vi "Process Monitor.vi"() -> ()   [LabVIEW 2016, in "SLL Process Monitor.lvlib"]
uses:
  SLL Process Monitor.lvlib
  <vilib>/Utility/error.llb/DialogType.ctl
  Source/SLL Queued State Machine/Queue Driver/Create Queue.vi
  Source/SLL Queued State Machine/Queue Driver/Enqueue an Item to Queue.vi
  Source/SLL Queued State Machine/Queue Driver/Dequeue Queue.vi
  Source/SLL Queued State Machine/Queue Driver/Enqueue N Items.vi
  Source/SLL Queued State Machine/Queue Driver/Flush Queue.vi
  Source/SLL Queued State Machine/Queue Driver/Release Queue.vi
  Source/SLL Queued State Machine/SLL QSM.lvlib
panel:
  in  "Sampling Rate (s)":dbl=1.0
  in  "Application Image Name":string="LabVIEW"
  out "Waveform Chart":T1(graph)
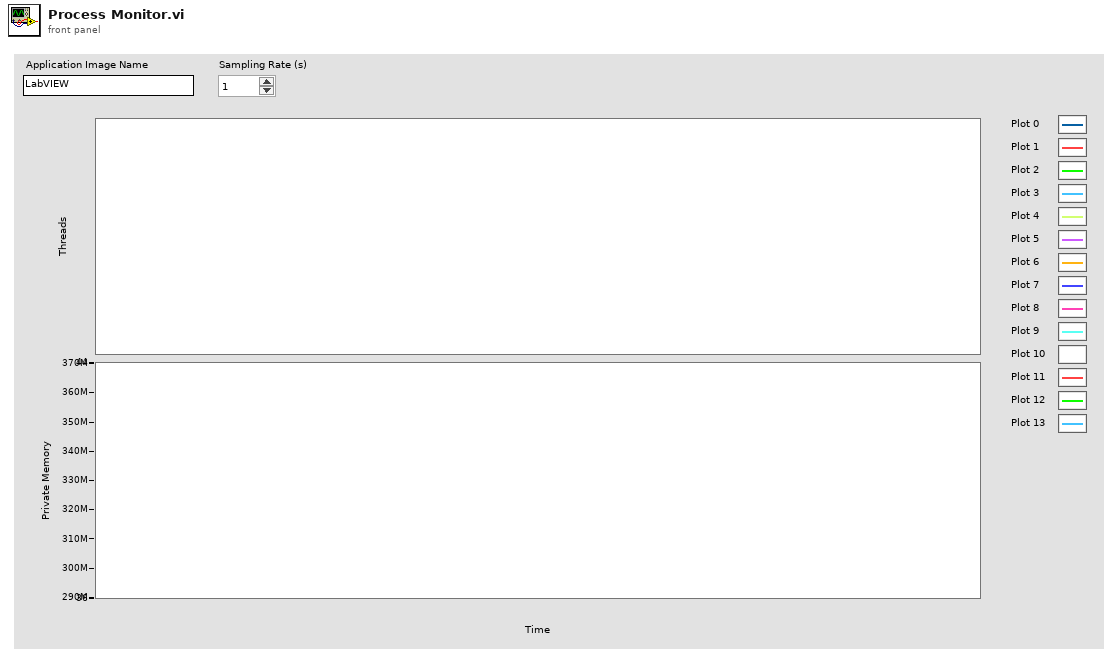
[diagram p1: front panel]
types:
  T1 = cluster{"Thread Count":i32, "PrivateMemorySize64":i64}
  T2 = cluster{"Flags":cluster{"Source Code?":bool}, "Application Name":string, "Ref":cluster{"ProcessMain":refnum<k24>, "UserProcess":refnum<k24>, "Threads":refnum<k24>}, "Sampling Rate (ms)":i32}
  T3 = cluster{"Thread Count":i32, "PrivateMemorySize64":i64}[]
  T4 = typedef "DialogType.ctl" = u16
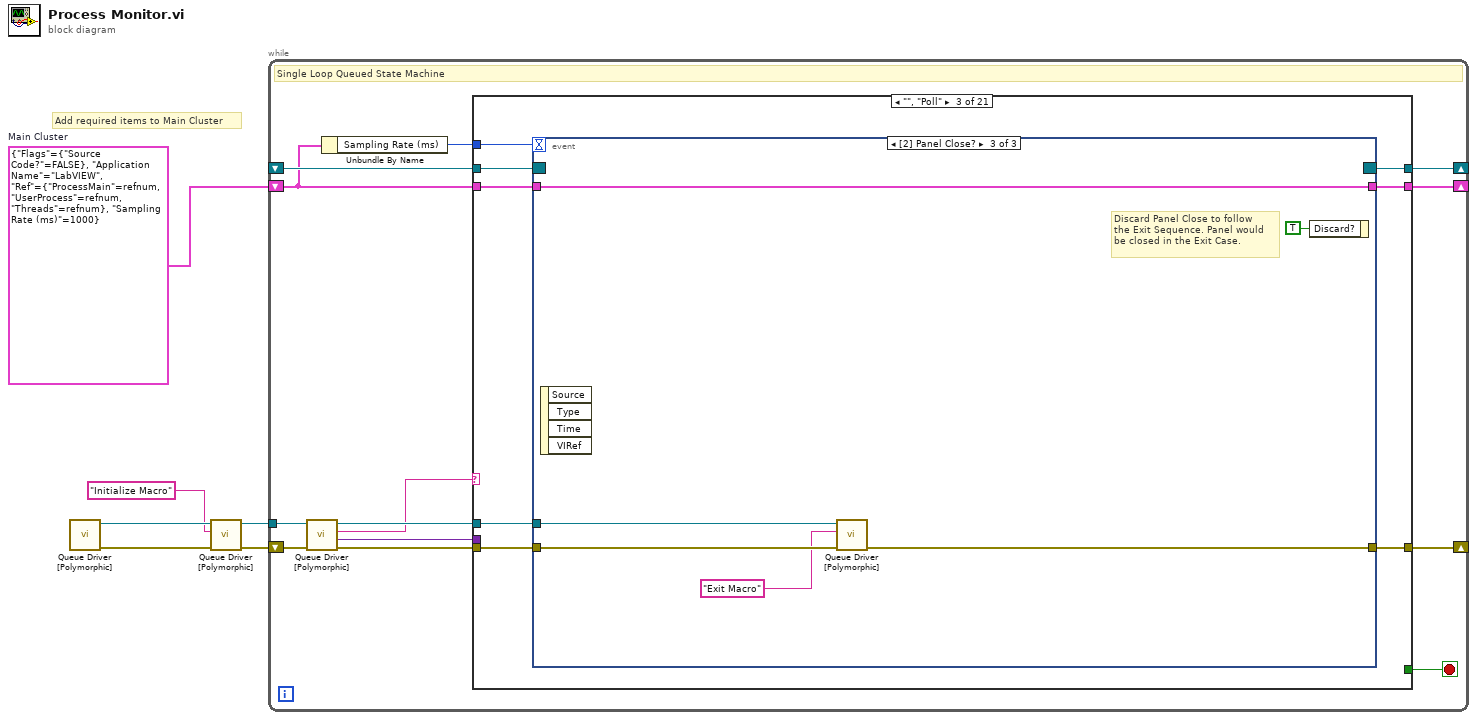
[diagram p0: block diagram]
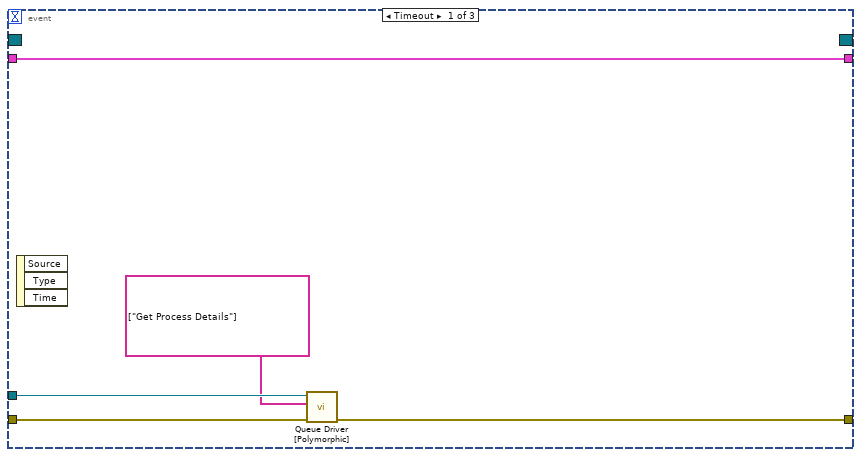
[diagram p4: hidden frame]
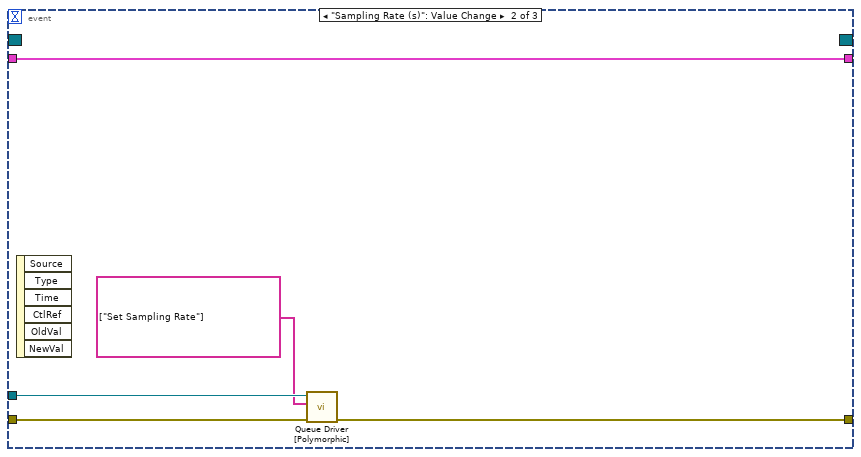
[diagram p5: hidden frame]
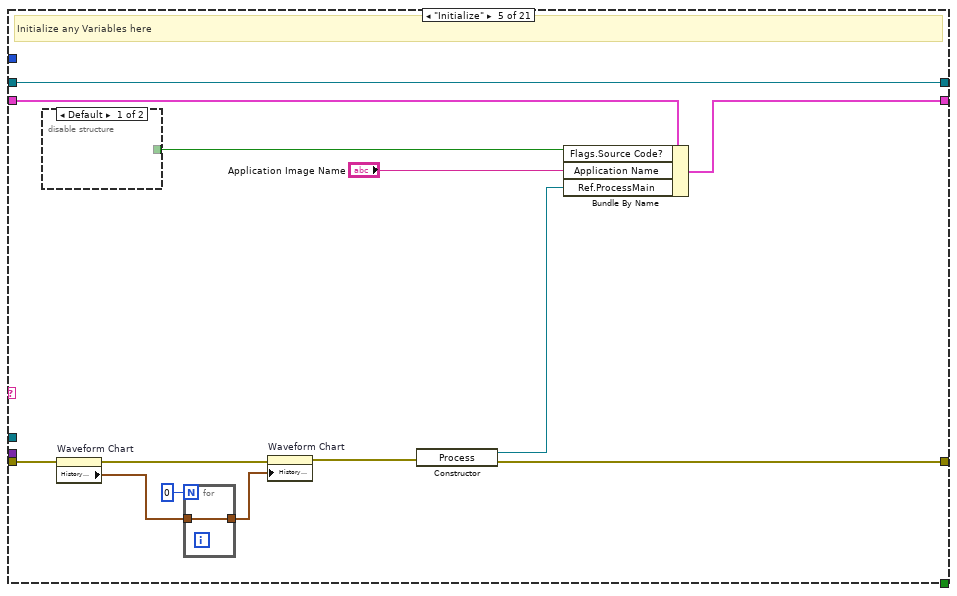
[diagram p7: hidden frame]
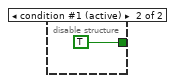
[diagram p8: hidden frame]
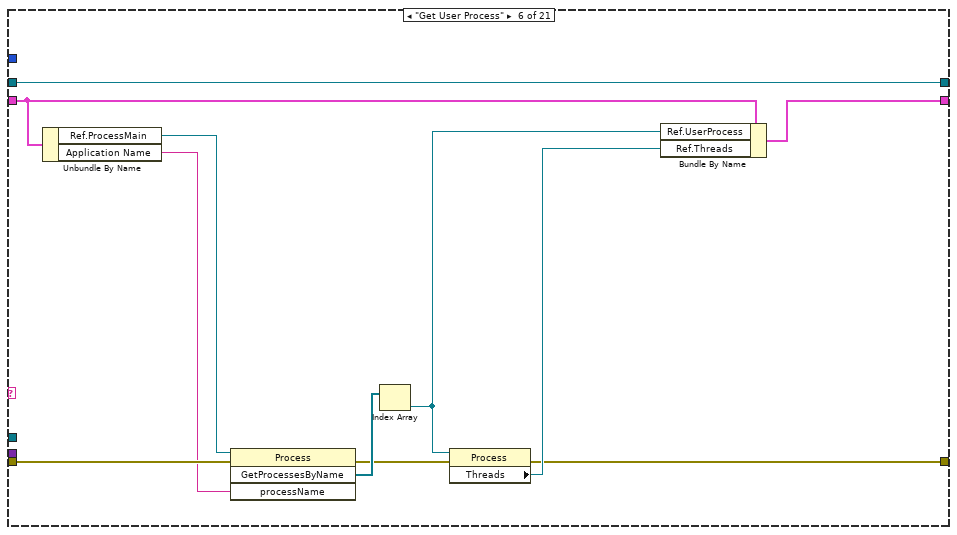
[diagram p9: hidden frame]
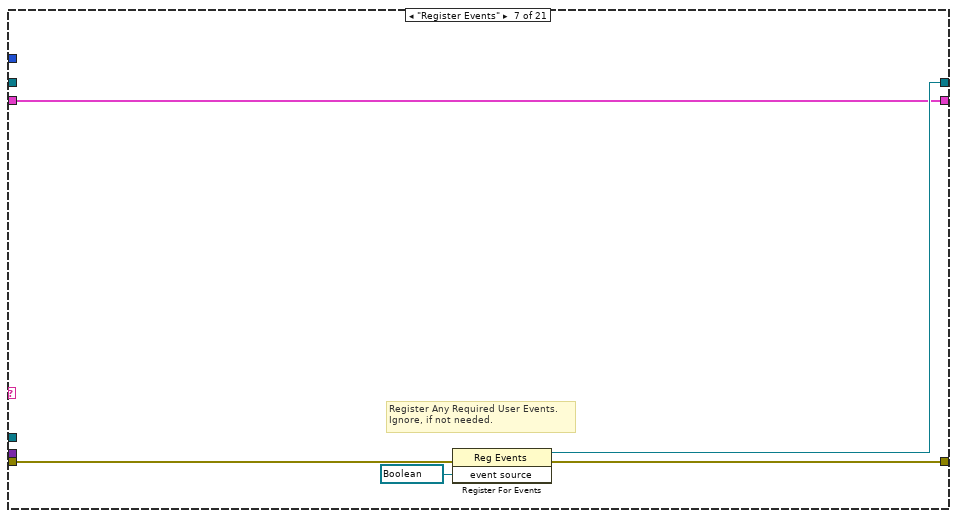
[diagram p10: hidden frame]
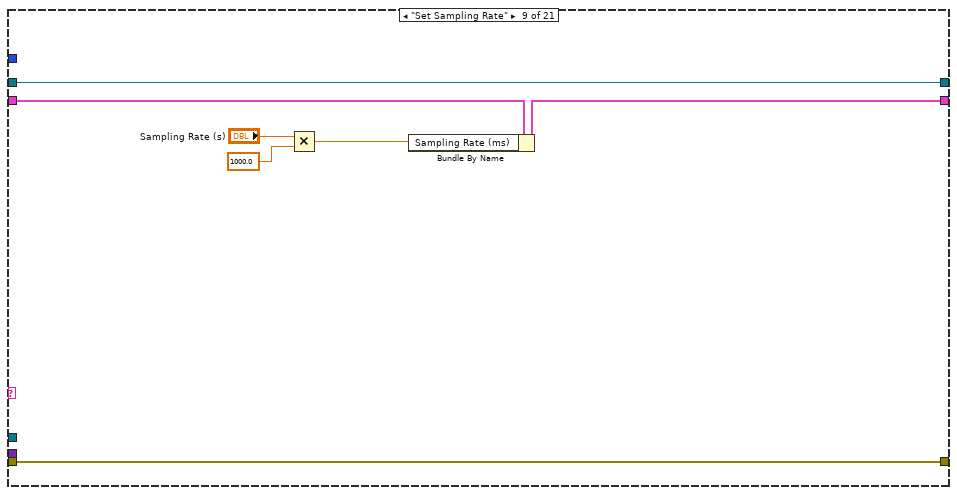
[diagram p12: hidden frame]
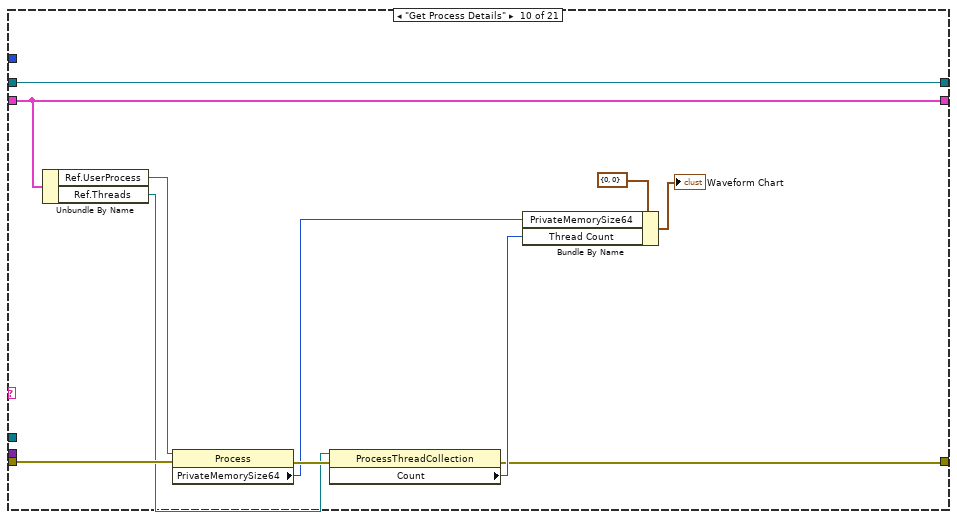
[diagram p13: hidden frame]
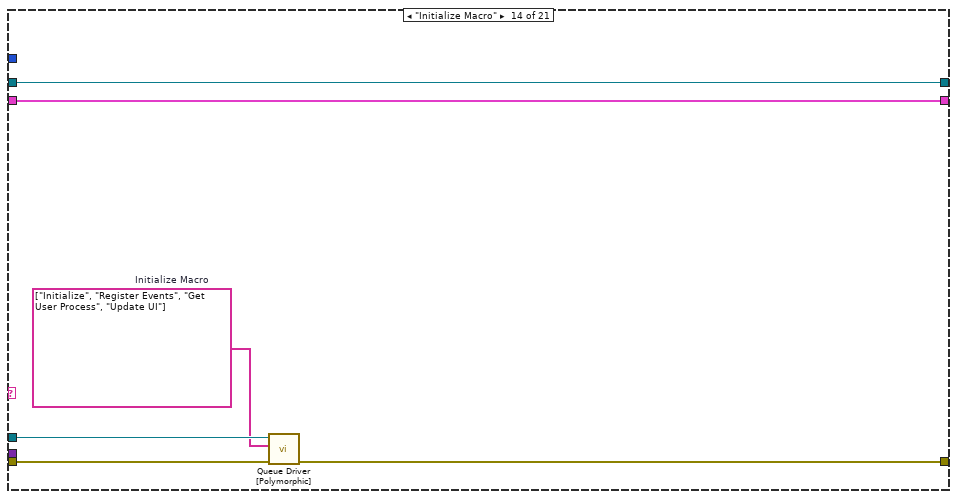
[diagram p17: hidden frame]
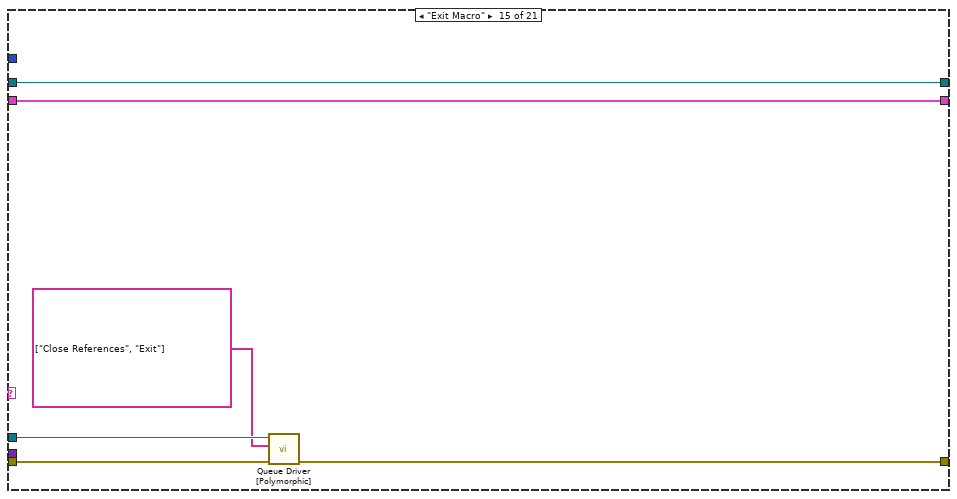
[diagram p18: hidden frame]
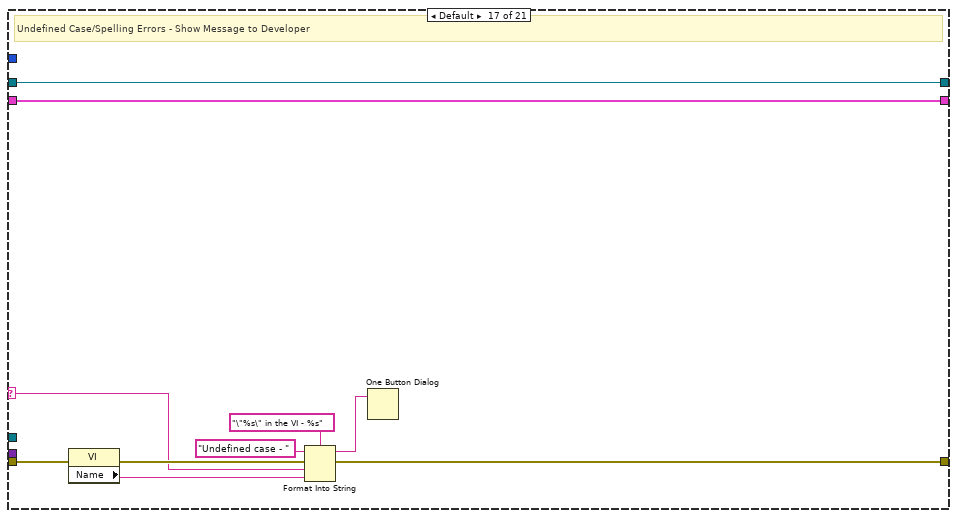
[diagram p20: hidden frame]
diagram:
  w6 = T2 {"Flags"={"Source Code?"=FALSE}, "Application Name"="LabVIEW", "Ref"={"ProcessMain"=refnum, "UserProcess"=refnum, "Threads"=refnum}, "Sampling Rate (ms)"=1000}  # Main Cluster
  # "Add required items to Main Cluster"
  n1 = call-poly "Queue Driver [Polymorphic].vi"() -> ("Error Out"=w4:errorcluster, "Queue Ref"=w3:refnum<queue>)  [unwired: 10 in]
  n2 = call-poly "Queue Driver [Polymorphic].vi"("Error In"=w4, "Item to Add"="Initialize Macro", "Queue Ref In"=w3) -> ("Error Out"=w5:errorcluster, "Queue Ref Out"=w1:refnum<queue>)  [unwired: 7 in]
  n3 = while "SLL Queued State Machine" {
    shift-right: [w17] -> _
    shift-left: w5 -> [w19]
    shift-right: [w14] -> _
    shift-left: _ -> [w13]
    shift-right: [w12] -> _
    shift-left: w6 -> [w10]
    tunnel: w1 -> [w8]
    stop <- w16 stop-if-true
    # "Single Loop Queued State Machine"
    n4 = call-poly "Queue Driver [Polymorphic].vi"("Error In"=w19, "Queue Ref In"=w8) -> ("Error Out"=w18:errorcluster, "Data"=w7:variant, "Dequeue"=w11:string, "Queue Ref Out"=w15:refnum<queue>)  [unwired: 6 in]
    n5 = Unbundle By Name(w10) -> ("Sampling Rate (ms)"=w9:i32)
    n6 = case "QSM Case Structure" shown="\"\", \"Poll\"" w11 {
      selector: w11 -> [_ _ _ _ _ _ _ _ _ _ _ _ _ _ _ _ w129 _ _ _ _]
      tunnel: w18 -> [w22 w25 w32 w52 w58 w75 w83 w86 w93 w102 w107 w110 w113 w117 w123 w128 w132 w144 w147 w149 w167]
      tunnel: [w22 w25 w33 w52 w60 w69 w82 w86 w93 w94 w107 w110 w113 w116 w122 w128 w135 w142 w147 w148 w163] -> w17
      tunnel: [_ _ _ _ _ _ _ _ _ _ _ _ _ _ _ _ _ _ _ _ TRUE] -> w16
      tunnel: [w21 w24 w31 w51 w65 w78 w81 w85 w92 w104 w106 w109 w112 w119 w125 w127 w138 w141 w146 w154 w166] -> w14
      tunnel: w13 -> [w21 w24 w30 w51 w65 w78 _ w85 w92 w104 w106 w109 w112 w119 w125 w127 w138 w141 w146 w154 w166]
      tunnel: [w20 w23 w28 w50 w62 w72 w80 w84 w88 w103 w105 w108 w111 w118 w124 w126 w137 w140 w145 w153 w165] -> w12
      tunnel: w10 -> [w20 w23 w29 w50 w63 w73 w80 w84 w91 w103 w105 w108 w111 w118 w124 w126 w137 w140 w145 w153 w165]
      tunnel: w9 -> [_ _ w27 _ _ _ _ _ _ _ _ _ _ _ _ _ _ _ _ _ _]
      tunnel: w15 -> [_ _ w26 _ _ _ _ _ _ _ _ _ _ w115 w121 _ _ _ _ _ w156]
      tunnel: w7 -> [_ _ _ _ _ _ _ _ _ _ _ _ _ _ _ _ _ _ _ _ _]
      frame "/--------------- Read Me -----------------/" {
        # "General Purpose Queue Based State Machine for Any Use Case (main application, module, pop up message etc)\n\nAdvantages:\n1. No Need to Pass Queue References between Queue Driver VIs.\n2. This template can be safely used in multiple parallel running modules without any issues.\n3. This template can also be safely used even in cases where the VI is configured to be a Clone, where multiple \ninstances of the VI could be executing concurrently.\n\nHow to Use:\n1. Add necessary items to the Main Cluster.\n2. Use the Polymorphic Queue Driver for doing any queue operations. There is no need to pass the queue driver\nreference, as the Queue Driver automatically infers the reference based on the VI instance from which it is called.\n3. Add any required user events in the \"Register Events\" case. Ignore if not needed.\n4. Use \"Sequences\" section for defining any list of state calls, which could be used in multiple places. \nEg: Initialize Sequence, might be needed if we need to any reinitialization."
      }
      frame "/------------------ Poll -------------------/" {
      }
      frame "", "Poll" {
        n7 = event shown="[2] Panel Close?" {
          selector: w30 -> [_ _ _]
          dyn-events: [_ _ _] -> w31
          timeout: w27 -> [_ _ _]
          tunnel: [w36 w41 w48] -> w33
          tunnel: w32 -> [w37 w42 w49]
          tunnel: w29 -> [w38 w43 w47]
          tunnel: [w38 w43 w47] -> w28
          tunnel: w26 -> [w35 w40 w44]
          event Timeout {
            n8 = event-data() -> ()  [unwired: 1 in, 3 out]
            n9 = call-poly "Queue Driver [Polymorphic].vi"("Error In"=w37, "Enqueue N"=string[] ["Get Process Details"], "Queue Ref In"=w35) -> ("Error Out"=w36:errorcluster)  [unwired: 7 in, 1 out]
          }
          event "Sampling Rate (s)": Value Change {
            n10 = event-data() -> ()  [unwired: 1 in, 6 out]
            n11 = call-poly "Queue Driver [Polymorphic].vi"("Error In"=w42, "Enqueue N"=string[] ["Set Sampling Rate"], "Queue Ref In"=w40) -> ("Error Out"=w41:errorcluster)  [unwired: 7 in, 1 out]
          }
          event Panel Close? {
            # "Discard Panel Close to follow\nthe Exit Sequence. Panel would\nbe closed in the Exit Case."
            n12 = event-data() -> ()  [unwired: 1 in, 4 out]
            n13 = call-poly "Queue Driver [Polymorphic].vi"("Error In"=w49, "Item to Add"="Exit Macro" ("Enqueue"), "Queue Ref In"=w44) -> ("Error Out"=w48:errorcluster)  [unwired: 7 in, 1 out]
            n14 = event-data("Discard?"=TRUE) -> ()  [unwired: 1 in, 1 out]
          }
        }
      }
      frame "/--------------- Initialize -----------------/" {
      }
      frame "Initialize" {
        # "Initialize any Variables here"
        n15 = disable-structure shown="Default" {
          disable-tunnel: [_ TRUE] -> w64
          frame condition #0 {
          }
          frame condition #1 (active) {
          }
        }
        n16 = property on="Waveform Chart" class="WFChart (strict)"(error in=w58) -> (error out=w57:errorcluster, "History Data"=w54:T3)  [unwired: 1 in, 1 out]
        n17 = for {
          N: 0 -> [_]
          tunnel: w54 -> [w66]
          tunnel: [w66] -> w53
        }
        n18 = property on="Waveform Chart" class="WFChart (strict)"(error in=w57, "History Data"=w53) -> (error out=w56:errorcluster)  [unwired: 1 in, 1 out]
        n19 = constructor class="Process"(error in=w56) -> (reference out=w59:refnum<k24>, error out=w60:errorcluster)  [unwired: 2 in, 1 out]
        n20 = Bundle By Name(cluster=w63, "Flags.Source Code?"=w64, "Application Name"="Application Image Name", "Ref.ProcessMain"=w59) -> (w62:T2)
      }
      frame "Get User Process" {
        n21 = Unbundle By Name(w73) -> ("Ref.ProcessMain"=w76:refnum<k24>, "Application Name"=w74:string)
        n22 = invoke class="Process" method="GetProcessesByName"(reference=w76, error in=w75, "processName"=w74) -> (error out=w68:errorcluster, "GetProcessesByName"=w77:refnum<k24>[])  [unwired: 1 in, 2 out]
        n23 = Index Array(array=w77) -> (element=w71:refnum<k24>)  [unwired: 1 in]
        n24 = property class="Process"(reference=w71, error in=w68) -> (error out=w69:errorcluster, "Threads"=w70:refnum<k24>)  [unwired: 1 out]
        n25 = Bundle By Name(cluster=w73, "Ref.UserProcess"=w71, "Ref.Threads"=w70) -> (w72:T2)
      }
      frame "Register Events" {
        # "Register Any Required User Events. \nIgnore, if not needed."
        n26 = register-events(error in=w83, refnum<vi> refnum ("event source")) -> (reference out=w81:refnum<event-registration>, error out=w82:errorcluster)  [unwired: 1 in]
      }
      frame "/---------- Process Monitor ----------/" {
      }
      frame "Set Sampling Rate" {
        n27 = Multiply(x="Sampling Rate (s)", y=1000.0) -> (x*y=w87:dbl)
        n28 = Bundle By Name(cluster=w91, "Sampling Rate (ms)"=w87) -> (w88:T2)
      }
      frame "Get Process Details" {
        n29 = Unbundle By Name(w103) -> ("Ref.UserProcess"=w101:refnum<k24>, "Ref.Threads"=w98:refnum<k24>)
        n30 = property class="Process"(reference=w101, error in=w102) -> (error out=w100:errorcluster, "PrivateMemorySize64"=w97:i64)  [unwired: 1 out]
        n31 = property class="ProcessThreadCollection"(reference=w98, error in=w100) -> (error out=w94:errorcluster, "Count"=w96:i32)  [unwired: 1 out]
        n32 = Bundle By Name(cluster=T1 {"Thread Count"=0, "PrivateMemorySize64"=0}, "PrivateMemorySize64"=w97, "Thread Count"=w96) -> (→"Waveform Chart":T1)
      }
      frame "/-------------- User Interface --------------/" {
        # "Duplicate this case to create additional case splitters for readability"
      }
      frame "Update UI" {
        # "Update Front Panel Controls in this Case"
      }
      frame "/----------------- Macros -----------------/" {
      }
      frame "Initialize Macro" {
        w114 = string[] ["Initialize", "Register Events", "Get User Process", "Update UI"]  # Initialize Macro
        n33 = call-poly "Queue Driver [Polymorphic].vi"("Error In"=w117, "Enqueue N"=w114, "Queue Ref In"=w115) -> ("Error Out"=w116:errorcluster)  [unwired: 7 in, 1 out]
      }
      frame "Exit Macro" {
        n34 = call-poly "Queue Driver [Polymorphic].vi"("Error In"=w123, "Enqueue N"=string[] ["Close References", "Exit"], "Queue Ref In"=w121) -> ("Error Out"=w122:errorcluster)  [unwired: 7 in, 1 out]
      }
      frame "/-------------- Error Handler--------------/" {
      }
      frame Default {
        # "Undefined Case/Spelling Errors - Show Message to Developer"
        n35 = property class="VI"(error in=w132) -> (error out=w131:errorcluster, "Name"=w130:string)  [unwired: 1 in, 1 out]
        n36 = Format Into String(format string="\"%s\" in the VI - %s" ("message"), initial string="Undefined case - ", error in=w131, w129, w130) -> (resulting string=w133:string, error out=w135:errorcluster)
        n37 = One Button Dialog(message=w133) -> ()  [unwired: 1 in, 1 out]
      }
      frame "Error" {
        w139 = T4 2 items=["no dialog", "OK message", "continue or stop message", "OK message + warnings", "continue/stop + warnings"] ("type of dialog (OK msg:1)")
        # "Handle the Error"
        n38 = call <vilib>:"Simple Error Handler.vi"("type of dialog (OK msg:1)"=w139, "error in (no error)"=w144) -> ("error out"=w143:errorcluster)  [unwired: 3 in, 4 out]
        n39 = call <vilib>:"Clear Errors.vi"("error in (no error)"=w143) -> ("error out"=w142:errorcluster)  [unwired: 5 in, 1 out]
      }
      frame "/------------------- Exit --------------------/" {
      }
      frame "Close References" {
        n40 = Unbundle By Name(w153) -> ("Ref.ProcessMain"=w150:refnum<k24>, "Ref.UserProcess"=w151:refnum<k24>)
        n41 = Close Reference(reference=w151, error in (no error)=w149) -> (error out=w152:errorcluster)
        n42 = Close Reference(reference=w150, error in (no error)=w152) -> (error out=w148:errorcluster)
      }
      frame "Exit" {
        n43 = call-poly "Queue Driver [Polymorphic].vi"("Error In"=w167, "Queue Ref In"=w156) -> ("Error Out"=w168:errorcluster, "Queue Ref Out"=w155:refnum<queue>)  [unwired: 7 in, 1 out]
        n44 = Unbundle By Name(w165) -> ("Flags.Source Code?"=w158:bool)
        n45 = call-poly "Queue Driver [Polymorphic].vi"("Error In"=w168, "Queue Ref In"=w155) -> ("Error Out"=w164:errorcluster)  [unwired: 9 in]
        n46 = Call Chain() -> (call chain=w162:string[])
        n47 = Array Size(array=w162) -> (size(s)=w161:i32)
        n48 = Equal?(x=w161, y=1) -> (x = y?=w159:bool)
        n49 = And(x=w158, y=w159) -> (x .and. y?=w157:bool)
        n50 = case "Skip Panel Close when in Source\nCode and is the top most caller" shown="True" w157 {
          tunnel: w164 -> [w171 w173]
          tunnel: [w172 w173] -> w163
          frame False {
            # "Close Panel"
            n51 = invoke class="VI" method="FP.Close"() -> (error out=w170:errorcluster)  [unwired: 3 in, 2 out]
            n52 = Merge Errors(w171, w170) -> (w172:errorcluster)
          }
          frame True {
            # "Do Not Close Panel"
          }
        }
      }
    }
  }
